vi "test TCX read (installed 71).vi"() -> ()   [LabVIEW 2011] (continued)
xmlns=\"http://www.garmin.com/xmlschemas/ActivityExtension/v2\"><Watts>70</Watts></TPX></Extensions></Trackpoint><Trackpoint><Time>2008-03-03T23:11:28Z</Time><Position><LatitudeDegrees>35.863362</LatitudeDegrees><LongitudeDegrees>-78.899874</LongitudeDegrees></Position><AltitudeMeters>78.004</AltitudeMeters><DistanceMeters>14315.783</DistanceMeters><Cadence>88</Cadence><Extensions><TPX xmlns=\"http://www.garmin.com/xmlschemas/ActivityExtension/v2\"><Watts>106</Watts></TPX></Extensions></Trackpoint><Trackpoint><Time>2008-03-03T23:11:29Z</Time><Position><LatitudeDegrees>35.863341</LatitudeDegrees><LongitudeDegrees>-78.900001</LongitudeDegrees></Position><AltitudeMeters>78.004</AltitudeMeters><DistanceMeters>14327.517</DistanceMeters><Cadence>89</Cadence><Extensions><TPX xmlns=\"http://www.garmin.com/xmlschemas/ActivityExtension/v2\"><Watts>108</Watts></TPX></Extensions></Trackpoint><Trackpoint><Time>2008-03-03T23:11:30Z</Time><Position><LatitudeDegrees>35.863322</LatitudeDegrees><LongitudeDegrees>-78.900129</LongitudeDegrees></Position><AltitudeMeters>77.523</AltitudeMeters><DistanceMeters>14339.211</DistanceMeters><Cadence>89</Cadence><Extensions><TPX xmlns=\"http://www.garmin.com/xmlschemas/ActivityExtension/v2\"><Watts>84</Watts></TPX></Extensions></Trackpoint><Trackpoint><Time>2008-03-03T23:11:31Z</Time><Position><LatitudeDegrees>35.863302</LatitudeDegrees><LongitudeDegrees>-78.900256</LongitudeDegrees></Position><AltitudeMeters>76.562</AltitudeMeters><DistanceMeters>14350.880</DistanceMeters><Cadence>88</Cadence><Extensions><TPX xmlns=\"http://www.garmin.com/xmlschemas/ActivityExtension/v2\"><Watts>71</Watts></TPX></Extensions></Trackpoint><Trackpoint><Time>2008-03-03T23:11:32Z</Time><Position><LatitudeDegrees>35.863280</LatitudeDegrees><LongitudeDegrees>-78.900379</LongitudeDegrees></Position><AltitudeMeters>76.562</AltitudeMeters><DistanceMeters>14362.324</DistanceMeters><Cadence>87</Cadence><Extensions><TPX xmlns=\"http://www.garmin.com/xmlschemas/ActivityExtension/v2\"><Watts>71</Watts></TPX></Extensions></Trackpoint><Trackpoint><Time>2008-03-03T23:11:33Z</Time><Position><LatitudeDegrees>35.863260</LatitudeDegrees><LongitudeDegrees>-78.900502</LongitudeDegrees></Position><AltitudeMeters>75.601</AltitudeMeters><DistanceMeters>14373.616</DistanceMeters><Cadence>86</Cadence><Extensions><TPX xmlns=\"http://www.garmin.com/xmlschemas/ActivityExtension/v2\"><Watts>86</Watts></TPX></Extensions></Trackpoint><Trackpoint><Time>2008-03-03T23:11:34Z</Time><Position><LatitudeDegrees>35.863238</LatitudeDegrees><LongitudeDegrees>-78.900622</LongitudeDegrees></Position><AltitudeMeters>75.601</AltitudeMeters><DistanceMeters>14384.671</DistanceMeters><Cadence>84</Cadence><Extensions><TPX xmlns=\"http://www.garmin.com/xmlschemas/ActivityExtension/v2\"><Watts>96</Watts></TPX></Extensions></Trackpoint><Trackpoint><Time>2008-03-03T23:11:35Z</Time><Position><LatitudeDegrees>35.863220</LatitudeDegrees><LongitudeDegrees>-78.900737</LongitudeDegrees></Position><AltitudeMeters>76.081</AltitudeMeters><DistanceMeters>14395.224</DistanceMeters><Cadence>81</Cadence><Extensions><TPX xmlns=\"http://www.garmin.com/xmlschemas/ActivityExtension/v2\"><Watts>97</Watts></TPX></Extensions></Trackpoint><Trackpoint><Time>2008-03-03T23:11:36Z</Time><Position><LatitudeDegrees>35.863205</LatitudeDegrees><LongitudeDegrees>-78.900847</LongitudeDegrees></Position><AltitudeMeters>75.601</AltitudeMeters><DistanceMeters>14405.182</DistanceMeters><Cadence>79</Cadence><Extensions><TPX xmlns=\"http://www.garmin.com/xmlschemas/ActivityExtension/v2\"><Watts>97</Watts></TPX></Extensions></Trackpoint><Trackpoint><Time>2008-03-03T23:11:37Z</Time><Position><LatitudeDegrees>35.863188</LatitudeDegrees><LongitudeDegrees>-78.900954</LongitudeDegrees></Position><AltitudeMeters>76.081</AltitudeMeters><DistanceMeters>14415.110</DistanceMeters><Cadence>75</Cadence><Extensions><TPX xmlns=\"http://www.garmin.com/xmlschemas/ActivityExtension/v2\"><Watts>109</Watts></TPX></Extensions></Trackpoint><Trackpoint><Time>2008-03-03T23:11:38Z</Time><Position><LatitudeDegrees>35.863172</LatitudeDegrees><LongitudeDegrees>-78.901058</LongitudeDegrees></Position><AltitudeMeters>76.081</AltitudeMeters><DistanceMeters>14424.662</DistanceMeters><Cadence>72</Cadence><Extensions><TPX xmlns=\"http://www.garmin.com/xmlschemas/ActivityExtension/v2\"><Watts>151</Watts></TPX></Extensions></Trackpoint><Trackpoint><Time>2008-03-03T23:11:39Z</Time><Position><LatitudeDegrees>35.863153</LatitudeDegrees><LongitudeDegrees>-78.901160</LongitudeDegrees></Position><AltitudeMeters>76.562</AltitudeMeters><DistanceMeters>14434.011</DistanceMeters><Cadence>72</Cadence><Extensions><TPX xmlns=\"http://www.garmin.com/xmlschemas/ActivityExtension/v2\"><Watts>152</Watts></TPX></Extensions></Trackpoint><Trackpoint><Time>2008-03-03T23:11:40Z</Time><Position><LatitudeDegrees>35.863133</LatitudeDegrees><LongitudeDegrees>-78.901258</LongitudeDegrees></Position><AltitudeMeters>77.043</AltitudeMeters><DistanceMeters>14443.188</DistanceMeters><Cadence>70</Cadence><Extensions><TPX xmlns=\"http://www.garmin.com/xmlschemas/ActivityExtension/v2\"><Watts>227</Watts></TPX></Extensions></Trackpoint><Trackpoint><Time>2008-03-03T23:11:41Z</Time><Position><LatitudeDegrees>35.863114</LatitudeDegrees><LongitudeDegrees>-78.901354</LongitudeDegrees></Position><AltitudeMeters>77.043</AltitudeMeters><DistanceMeters>14452.078</DistanceMeters><Cadence>68</Cadence><Extensions><TPX xmlns=\"http://www.garmin.com/xmlschemas/ActivityExtension/v2\"><Watts>274</Watts></TPX></Extensions></Trackpoint><Trackpoint><Time>2008-03-03T23:11:42Z</Time><Position><LatitudeDegrees>35.863093</LatitudeDegrees><LongitudeDegrees>-78.901448</LongitudeDegrees></Position><AltitudeMeters>77.043</AltitudeMeters><DistanceMeters>14460.851</DistanceMeters><Cadence>67</Cadence><Extensions><TPX xmlns=\"http://www.garmin.com/xmlschemas/ActivityExtension/v2\"><Watts>260</Watts></TPX></Extensions></Trackpoint><Trackpoint><Time>2008-03-03T23:11:43Z</Time><Position><LatitudeDegrees>35.863073</LatitudeDegrees><LongitudeDegrees>-78.901541</LongitudeDegrees></Position><AltitudeMeters>77.043</AltitudeMeters><DistanceMeters>14469.592</DistanceMeters><Cadence>67</Cadence><Extensions><TPX xmlns=\"http://www.garmin.com/xmlschemas/ActivityExtension/v2\"><Watts>261</Watts></TPX></Extensions></Trackpoint><Trackpoint><Time>2008-03-03T23:11:44Z</Time><Position><LatitudeDegrees>35.863051</LatitudeDegrees><LongitudeDegrees>-78.901635</LongitudeDegrees></Position><AltitudeMeters>77.043</AltitudeMeters><DistanceMeters>14478.395</DistanceMeters><Cadence>66</Cadence><Extensions><TPX xmlns=\"http://www.garmin.com/xmlschemas/ActivityExtension/v2\"><Watts>229</Watts></TPX></Extensions></Trackpoint><Trackpoint><Time>2008-03-03T23:11:45Z</Time><Position><LatitudeDegrees>35.863029</LatitudeDegrees><LongitudeDegrees>-78.901729</LongitudeDegrees></Position><AltitudeMeters>78.004</AltitudeMeters><DistanceMeters>14487.213</DistanceMeters><Cadence>67</Cadence><Extensions><TPX xmlns=\"http://www.garmin.com/xmlschemas/ActivityExtension/v2\"><Watts>209</Watts></TPX></Extensions></Trackpoint><Trackpoint><Time>2008-03-03T23:11:46Z</Time><Position><LatitudeDegrees>35.863005</LatitudeDegrees><LongitudeDegrees>-78.901822</LongitudeDegrees></Position><AltitudeMeters>78.004</AltitudeMeters><DistanceMeters>14496.032</DistanceMeters><Cadence>67</Cadence><Extensions><TPX xmlns=\"http://www.garmin.com/xmlschemas/ActivityExtension/v2\"><Watts>201</Watts></TPX></Extensions></Trackpoint><Trackpoint><Time>2008-03-03T23:11:47Z</Time><Position><LatitudeDegrees>35.862982</LatitudeDegrees><LongitudeDegrees>-78.901916</LongitudeDegrees></Position><AltitudeMeters>78.004</AltitudeMeters><DistanceMeters>14504.937</DistanceMeters><Cadence>68</Cadence><Extensions><TPX xmlns=\"http://www.garmin.com/xmlschemas/ActivityExtension/v2\"><Watts>202</Watts></TPX></Extensions></Trackpoint><Trackpoint><Time>2008-03-03T23:11:48Z</Time><Position><LatitudeDegrees>35.862958</LatitudeDegrees><LongitudeDegrees>-78.902011</LongitudeDegrees></Position><AltitudeMeters>77.523</AltitudeMeters><DistanceMeters>14513.910</DistanceMeters><Cadence>69</Cadence><Extensions><TPX xmlns=\"http://www.garmin.com/xmlschemas/ActivityExtension/v2\"><Watts>197</Watts></TPX></Extensions></Trackpoint><Trackpoint><Time>2008-03-03T23:11:49Z</Time><Position><LatitudeDegrees>35.862929</LatitudeDegrees><LongitudeDegrees>-78.902105</LongitudeDegrees></Position><AltitudeMeters>77.523</AltitudeMeters><DistanceMeters>14523.009</DistanceMeters><Cadence>69</Cadence><Extensions><TPX xmlns=\"http://www.garmin.com/xmlschemas/ActivityExtension/v2\"><Watts>197</Watts></TPX></Extensions></Trackpoint><Trackpoint><Time>2008-03-03T23:11:50Z</Time><Position><LatitudeDegrees>35.862900</LatitudeDegrees><LongitudeDegrees>-78.902200</LongitudeDegrees></Position><AltitudeMeters>78.004</AltitudeMeters><DistanceMeters>14532.178</DistanceMeters><Cadence>69</Cadence><Extensions><TPX xmlns=\"http://www.garmin.com/xmlschemas/ActivityExtension/v2\"><Watts>192</Watts></TPX></Extensions></Trackpoint><Trackpoint><Time>2008-03-03T23:11:51Z</Time><Position><LatitudeDegrees>35.862869</LatitudeDegrees><LongitudeDegrees>-78.902294</LongitudeDegrees></Position><AltitudeMeters>77.043</AltitudeMeters><DistanceMeters>14541.325</DistanceMeters><Cadence>69</Cadence><Extensions><TPX xmlns=\"http://www.garmin.com/xmlschemas/ActivityExtension/v2\"><Watts>192</Watts></TPX></Extensions></Trackpoint><Trackpoint><Time>2008-03-03T23:11:52Z</Time><Position><LatitudeDegrees>35.862839</LatitudeDegrees><LongitudeDegrees>-78.902389</LongitudeDegrees></Position><AltitudeMeters>76.562</AltitudeMeters><DistanceMeters>14550.554</DistanceMeters><Cadence>70</Cadence><Extensions><TPX xmlns=\"http://www.garmin.com/xmlschemas/ActivityExtension/v2\"><Watts>177</Watts></TPX></Extensions></Trackpoint><Trackpoint><Time>2008-03-03T23:11:53Z</Time><Position><LatitudeDegrees>35.862807</LatitudeDegrees><LongitudeDegrees>-78.902486</LongitudeDegrees></Position><AltitudeMeters>77.043</AltitudeMeters><DistanceMeters>14559.941</DistanceMeters><Cadence>71</Cadence><Extensions><TPX xmlns=\"http://www.garmin.com/xmlschemas/ActivityExtension/v2\"><Watts>164</Watts></TPX></Extensions></Trackpoint><Trackpoint><Time>2008-03-03T23:11:54Z</Time><Position><LatitudeDegrees>35.862774</LatitudeDegrees><LongitudeDegrees>-78.902581</LongitudeDegrees></Position><AltitudeMeters>76.562</AltitudeMeters><DistanceMeters>14569.321</DistanceMeters><Cadence>71</Cadence><Extensions><TPX xmlns=\"http://www.garmin.com/xmlschemas/ActivityExtension/v2\"><Watts>150</Watts></TPX></Extensions></Trackpoint><Trackpoint><Time>2008-03-03T23:11:55Z</Time><Position><LatitudeDegrees>35.862742</LatitudeDegrees><LongitudeDegrees>-78.902678</LongitudeDegrees></Position><AltitudeMeters>76.562</AltitudeMeters><DistanceMeters>14578.787</DistanceMeters><Cadence>72</Cadence><Extensions><TPX xmlns=\"http://www.garmin.com/xmlschemas/ActivityExtension/v2\"><Watts>137</Watts></TPX></Extensions></Trackpoint><Trackpoint><Time>2008-03-03T23:11:56Z</Time><Position><LatitudeDegrees>35.862709</LatitudeDegrees><LongitudeDegrees>-78.902777</LongitudeDegrees></Position><AltitudeMeters>76.081</AltitudeMeters><DistanceMeters>14588.439</DistanceMeters><Cadence>72</Cadence><Extensions><TPX xmlns=\"http://www.garmin.com/xmlschemas/ActivityExtension/v2\"><Watts>136</Watts></TPX></Extensions></Trackpoint><Trackpoint><Time>2008-03-03T23:11:57Z</Time><Position><LatitudeDegrees>35.862676</LatitudeDegrees><LongitudeDegrees>-78.902876</LongitudeDegrees></Position><AltitudeMeters>76.081</AltitudeMeters><DistanceMeters>14598.146</DistanceMeters><Cadence>74</Cadence><Extensions><TPX xmlns=\"http://www.garmin.com/xmlschemas/ActivityExtension/v2\"><Watts>129</Watts></TPX></Extensions></Trackpoint><Trackpoint><Time>2008-03-03T23:11:58Z</Time><Position><LatitudeDegrees>35.862642</LatitudeDegrees><LongitudeDegrees>-78.902977</LongitudeDegrees></Position><AltitudeMeters>76.081</AltitudeMeters><DistanceMeters>14607.972</DistanceMeters><Cadence>74</Cadence><Extensions><TPX xmlns=\"http://www.garmin.com/xmlschemas/ActivityExtension/v2\"><Watts>128</Watts></TPX></Extensions></Trackpoint><Trackpoint><Time>2008-03-03T23:11:59Z</Time><Position><LatitudeDegrees>35.862609</LatitudeDegrees><LongitudeDegrees>-78.903079</LongitudeDegrees></Position><AltitudeMeters>75.601</AltitudeMeters><DistanceMeters>14617.938</DistanceMeters><Cadence>76</Cadence><Extensions><TPX xmlns=\"http://www.garmin.com/xmlschemas/ActivityExtension/v2\"><Watts>102</Watts></TPX></Extensions></Trackpoint><Trackpoint><Time>2008-03-03T23:12:00Z</Time><Position><LatitudeDegrees>35.862574</LatitudeDegrees><LongitudeDegrees>-78.903183</LongitudeDegrees></Position><AltitudeMeters>75.601</AltitudeMeters><DistanceMeters>14628.073</DistanceMeters><Cadence>77</Cadence><Extensions><TPX xmlns=\"http://www.garmin.com/xmlschemas/ActivityExtension/v2\"><Watts>87</Watts></TPX></Extensions></Trackpoint><Trackpoint><Time>2008-03-03T23:12:01Z</Time><Position><LatitudeDegrees>35.862540</LatitudeDegrees><LongitudeDegrees>-78.903288</LongitudeDegrees></Position><AltitudeMeters>75.601</AltitudeMeters><DistanceMeters>14638.298</DistanceMeters><Cadence>77</Cadence><Extensions><TPX xmlns=\"http://www.garmin.com/xmlschemas/ActivityExtension/v2\"><Watts>87</Watts></TPX></Extensions></Trackpoint><Trackpoint><Time>2008-03-03T23:12:02Z</Time><Position><LatitudeDegrees>35.862505</LatitudeDegrees><LongitudeDegrees>-78.903394</LongitudeDegrees></Position><AltitudeMeters>75.601</AltitudeMeters><DistanceMeters>14648.685</DistanceMeters><Cadence>78</Cadence><Extensions><TPX xmlns=\"http://www.garmin.com/xmlschemas/ActivityExtension/v2\"><Watts>87</Watts></TPX></Extensions></Trackpoint><Trackpoint><Time>2008-03-03T23:12:03Z</Time><Position><LatitudeDegrees>35.862470</LatitudeDegrees><LongitudeDegrees>-78.903503</LongitudeDegrees></Position><AltitudeMeters>75.120</AltitudeMeters><DistanceMeters>14659.182</DistanceMeters><Cadence>79</Cadence><Extensions><TPX xmlns=\"http://www.garmin.com/xmlschemas/ActivityExtension/v2\"><Watts>87</Watts></TPX></Extensions></Trackpoint><Trackpoint><Time>2008-03-03T23:12:04Z</Time><Position><LatitudeDegrees>35.862435</LatitudeDegrees><LongitudeDegrees>-78.903612</LongitudeDegrees></Position><AltitudeMeters>74.640</AltitudeMeters><DistanceMeters>14669.802</DistanceMeters><Cadence>80</Cadence><Extensions><TPX xmlns=\"http://www.garmin.com/xmlschemas/ActivityExtension/v2\"><Watts>93</Watts></TPX></Extensions></Trackpoint><Trackpoint><Time>2008-03-03T23:12:05Z</Time><Position><LatitudeDegrees>35.862398</LatitudeDegrees><LongitudeDegrees>-78.903722</LongitudeDegrees></Position><AltitudeMeters>73.678</AltitudeMeters><DistanceMeters>14680.509</DistanceMeters><Cadence>81</Cadence><Extensions><TPX xmlns=\"http://www.garmin.com/xmlschemas/ActivityExtension/v2\"><Watts>94</Watts></TPX></Extensions></Trackpoint><Trackpoint><Time>2008-03-03T23:12:06Z</Time><Position><LatitudeDegrees>35.862362</LatitudeDegrees><LongitudeDegrees>-78.903832</LongitudeDegrees></Position><AltitudeMeters>73.198</AltitudeMeters><DistanceMeters>14691.294</DistanceMeters><Cadence>82</Cadence><Extensions><TPX xmlns=\"http://www.garmin.com/xmlschemas/ActivityExtension/v2\"><Watts>92</Watts></TPX></Extensions></Trackpoint><Trackpoint><Time>2008-03-03T23:12:07Z</Time><Position><LatitudeDegrees>35.862326</LatitudeDegrees><LongitudeDegrees>-78.903942</LongitudeDegrees></Position><AltitudeMeters>73.198</AltitudeMeters><DistanceMeters>14702.009</DistanceMeters><Cadence>81</Cadence><Extensions><TPX xmlns=\"http://www.garmin.com/xmlschemas/ActivityExtension/v2\"><Watts>97</Watts></TPX></Extensions></Trackpoint><Trackpoint><Time>2008-03-03T23:12:08Z</Time><Position><LatitudeDegrees>35.862289</LatitudeDegrees><LongitudeDegrees>-78.904050</LongitudeDegrees></Position><AltitudeMeters>73.678</AltitudeMeters><DistanceMeters>14712.588</DistanceMeters><Cadence>80</Cadence><Extensions><TPX xmlns=\"http://www.garmin.com/xmlschemas/ActivityExtension/v2\"><Watts>97</Watts></TPX></Extensions></Trackpoint><Trackpoint><Time>2008-03-03T23:12:09Z</Time><Position><LatitudeDegrees>35.862253</LatitudeDegrees><LongitudeDegrees>-78.904157</LongitudeDegrees></Position><AltitudeMeters>73.198</AltitudeMeters><DistanceMeters>14723.039</DistanceMeters><Cadence>79</Cadence><Extensions><TPX xmlns=\"http://www.garmin.com/xmlschemas/ActivityExtension/v2\"><Watts>125</Watts></TPX></Extensions></Trackpoint><Trackpoint><Time>2008-03-03T23:12:10Z</Time><Position><LatitudeDegrees>35.862219</LatitudeDegrees><LongitudeDegrees>-78.904263</LongitudeDegrees></Position><AltitudeMeters>73.678</AltitudeMeters><DistanceMeters>14733.320</DistanceMeters><Cadence>79</Cadence><Extensions><TPX xmlns=\"http://www.garmin.com/xmlschemas/ActivityExtension/v2\"><Watts>124</Watts></TPX></Extensions></Trackpoint><Trackpoint><Time>2008-03-03T23:12:11Z</Time><Position><LatitudeDegrees>35.862188</LatitudeDegrees><LongitudeDegrees>-78.904368</LongitudeDegrees></Position><AltitudeMeters>73.678</AltitudeMeters><DistanceMeters>14743.404</DistanceMeters><Cadence>77</Cadence><Extensions><TPX xmlns=\"http://www.garmin.com/xmlschemas/ActivityExtension/v2\"><Watts>144</Watts></TPX></Extensions></Trackpoint><Trackpoint><Time>2008-03-03T23:12:12Z</Time><Position><LatitudeDegrees>35.862162</LatitudeDegrees><LongitudeDegrees>-78.904473</LongitudeDegrees></Position><AltitudeMeters>74.159</AltitudeMeters><DistanceMeters>14753.264</DistanceMeters><Cadence>73</Cadence><Extensions><TPX xmlns=\"http://www.garmin.com/xmlschemas/ActivityExtension/v2\"><Watts>176</Watts></TPX></Extensions></Trackpoint><Trackpoint><Time>2008-03-03T23:12:13Z</Time><Position><LatitudeDegrees>35.862142</LatitudeDegrees><LongitudeDegrees>-78.904576</LongitudeDegrees></Position><AltitudeMeters>74.640</AltitudeMeters><DistanceMeters>14762.778</DistanceMeters><Cadence>73</Cadence><Extensions><TPX xmlns=\"http://www.garmin.com/xmlschemas/ActivityExtension/v2\"><Watts>176</Watts></TPX></Extensions></Trackpoint><Trackpoint><Time>2008-03-03T23:12:14Z</Time><Position><LatitudeDegrees>35.862129</LatitudeDegrees><LongitudeDegrees>-78.904676</LongitudeDegrees></Position><AltitudeMeters>75.120</AltitudeMeters><DistanceMeters>14771.976</DistanceMeters><Cadence>69</Cadence><Extensions><TPX xmlns=\"http://www.garmin.com/xmlschemas/ActivityExtension/v2\"><Watts>178</Watts></TPX></Extensions></Trackpoint><Trackpoint><Time>2008-03-03T23:12:15Z</Time><Position><LatitudeDegrees>35.862125</LatitudeDegrees><LongitudeDegrees>-78.904774</LongitudeDegrees></Position><AltitudeMeters>75.120</AltitudeMeters><DistanceMeters>14780.801</DistanceMeters><Cadence>67</Cadence><Extensions><TPX xmlns=\"http://www.garmin.com/xmlschemas/ActivityExtension/v2\"><Watts>180</Watts></TPX></Extensions></Trackpoint><Trackpoint><Time>2008-03-03T23:12:16Z</Time><Position><LatitudeDegrees>35.862130</LatitudeDegrees><LongitudeDegrees>-78.904870</LongitudeDegrees></Position><AltitudeMeters>75.601</AltitudeMeters><DistanceMeters>14789.530</DistanceMeters><Cadence>66</Cadence><Extensions><TPX xmlns=\"http://www.garmin.com/xmlschemas/ActivityExtension/v2\"><Watts>190</Watts></TPX></Extensions></Trackpoint><Trackpoint><Time>2008-03-03T23:12:17Z</Time><Position><LatitudeDegrees>35.862142</LatitudeDegrees><LongitudeDegrees>-78.904963</LongitudeDegrees></Position><AltitudeMeters>75.601</AltitudeMeters><DistanceMeters>14797.981</DistanceMeters><Cadence>66</Cadence><Extensions><TPX xmlns=\"http://www.garmin.com/xmlschemas/ActivityExtension/v2\"><Watts>192</Watts></TPX></Extensions></Trackpoint><Trackpoint><Time>2008-03-03T23:12:18Z</Time><Position><LatitudeDegrees>35.862161</LatitudeDegrees><LongitudeDegrees>-78.905054</LongitudeDegrees></Position><AltitudeMeters>75.601</AltitudeMeters><DistanceMeters>14806.480</DistanceMeters><Cadence>66</Cadence><Extensions><TPX xmlns=\"http://www.garmin.com/xmlschemas/ActivityExtension/v2\"><Watts>191</Watts></TPX></Extensions></Trackpoint><Trackpoint><Time>2008-03-03T23:12:19Z</Time><Position><LatitudeDegrees>35.862188</LatitudeDegrees><LongitudeDegrees>-78.905144</LongitudeDegrees></Position><AltitudeMeters>74.640</AltitudeMeters><DistanceMeters>14815.028</DistanceMeters><Cadence>66</Cadence><Extensions><TPX xmlns=\"http://www.garmin.com/xmlschemas/ActivityExtension/v2\"><Watts>185</Watts></TPX></Extensions></Trackpoint><Trackpoint><Time>2008-03-03T23:12:20Z</Time><Position><LatitudeDegrees>35.862220</LatitudeDegrees><LongitudeDegrees>-78.905230</LongitudeDegrees></Position><AltitudeMeters>74.640</AltitudeMeters><DistanceMeters>14823.684</DistanceMeters><Cadence>66</Cadence><Extensions><TPX xmlns=\"http://www.garmin.com/xmlschemas/ActivityExtension/v2\"><Watts>183</Watts></TPX></Extensions></Trackpoint><Trackpoint><Time>2008-03-03T23:12:21Z</Time><Position><LatitudeDegrees>35.862256</LatitudeDegrees><LongitudeDegrees>-78.905316</LongitudeDegrees></Position><AltitudeMeters>74.159</AltitudeMeters><DistanceMeters>14832.372</DistanceMeters><Cadence>67</Cadence><Extensions><TPX xmlns=\"http://www.garmin.com/xmlschemas/ActivityExtension/v2\"><Watts>179</Watts></TPX></Extensions></Trackpoint><Trackpoint><Time>2008-03-03T23:12:22Z</Time><Position><LatitudeDegrees>35.862293</LatitudeDegrees><LongitudeDegrees>-78.905401</LongitudeDegrees></Position><AltitudeMeters>74.159</AltitudeMeters><DistanceMeters>14841.090</DistanceMeters><Cadence>67</Cadence><Extensions><TPX xmlns=\"http://www.garmin.com/xmlschemas/ActivityExtension/v2\"><Watts>168</Watts></TPX></Extensions></Trackpoint><Trackpoint><Time>2008-03-03T23:12:23Z</Time><Position><LatitudeDegrees>35.862330</LatitudeDegrees><LongitudeDegrees>-78.905486</LongitudeDegrees></Position><AltitudeMeters>74.159</AltitudeMeters><DistanceMeters>14849.768</DistanceMeters><Cadence>66</Cadence><Extensions><TPX xmlns=\"http://www.garmin.com/xmlschemas/ActivityExtension/v2\"><Watts>170</Watts></TPX></Extensions></Trackpoint><Trackpoint><Time>2008-03-03T23:12:24Z</Time><Position><LatitudeDegrees>35.862367</LatitudeDegrees><LongitudeDegrees>-78.905570</LongitudeDegrees></Position><AltitudeMeters>74.159</AltitudeMeters><DistanceMeters>14858.395</DistanceMeters><Cadence>66</Cadence><Extensions><TPX xmlns=\"http://www.garmin.com/xmlschemas/ActivityExtension/v2\"><Watts>173</Watts></TPX></Extensions></Trackpoint><Trackpoint><Time>2008-03-03T23:12:25Z</Time><Position><LatitudeDegrees>35.862405</LatitudeDegrees><LongitudeDegrees>-78.905651</LongitudeDegrees></Position><AltitudeMeters>74.640</AltitudeMeters><DistanceMeters>14866.879</DistanceMeters><Cadence>65</Cadence><Extensions><TPX xmlns=\"http://www.garmin.com/xmlschemas/ActivityExtension/v2\"><Watts>169</Watts></TPX></Extensions></Trackpoint><Trackpoint><Time>2008-03-03T23:12:26Z</Time><Position><LatitudeDegrees>35.862443</LatitudeDegrees><LongitudeDegrees>-78.905731</LongitudeDegrees></Position><AltitudeMeters>74.640</AltitudeMeters><DistanceMeters>14875.242</DistanceMeters><Cadence>68</Cadence><Extensions><TPX xmlns=\"http://www.garmin.com/xmlschemas/ActivityExtension/v2\"><Watts>164</Watts></TPX></Extensions></Trackpoint><Trackpoint><Time>2008-03-03T23:12:27Z</Time><Position><LatitudeDegrees>35.862480</LatitudeDegrees><LongitudeDegrees>-78.905811</LongitudeDegrees></Position><AltitudeMeters>74.640</AltitudeMeters><DistanceMeters>14883.440</DistanceMeters><Cadence>76</Cadence><Extensions><TPX xmlns=\"http://www.garmin.com/xmlschemas/ActivityExtension/v2\"><Watts>171</Watts></TPX></Extensions></Trackpoint><Trackpoint><Time>2008-03-03T23:12:28Z</Time><Position><LatitudeDegrees>35.862514</LatitudeDegrees><LongitudeDegrees>-78.905888</LongitudeDegrees></Position><AltitudeMeters>75.120</AltitudeMeters><DistanceMeters>14891.395</DistanceMeters><Cadence>74</Cadence><Extensions><TPX xmlns=\"http://www.garmin.com/xmlschemas/ActivityExtension/v2\"><Watts>183</Watts></TPX></Extensions></Trackpoint><Trackpoint><Time>2008-03-03T23:12:29Z</Time><Position><LatitudeDegrees>35.862548</LatitudeDegrees><LongitudeDegrees>-78.905964</LongitudeDegrees></Position><AltitudeMeters>75.120</AltitudeMeters><DistanceMeters>14899.225</DistanceMeters><Cadence>72</Cadence><Extensions><TPX xmlns=\"http://www.garmin.com/xmlschemas/ActivityExtension/v2\"><Watts>260</Watts></TPX></Extensions></Trackpoint><Trackpoint><Time>2008-03-03T23:12:30Z</Time><Position><LatitudeDegrees>35.862580</LatitudeDegrees><LongitudeDegrees>-78.906040</LongitudeDegrees></Position><AltitudeMeters>75.601</AltitudeMeters><DistanceMeters>14906.950</DistanceMeters><Cadence>72</Cadence><Extensions><TPX xmlns=\"http://www.garmin.com/xmlschemas/ActivityExtension/v2\"><Watts>302</Watts></TPX></Extensions></Trackpoint><Trackpoint><Time>2008-03-03T23:12:31Z</Time><Position><LatitudeDegrees>35.862613</LatitudeDegrees><LongitudeDegrees>-78.906115</LongitudeDegrees></Position><AltitudeMeters>76.081</AltitudeMeters><DistanceMeters>14914.627</DistanceMeters><Cadence>72</Cadence><Extensions><TPX xmlns=\"http://www.garmin.com/xmlschemas/ActivityExtension/v2\"><Watts>337</Watts></TPX></Extensions></Trackpoint><Trackpoint><Time>2008-03-03T23:12:32Z</Time><Position><LatitudeDegrees>35.862646</LatitudeDegrees><LongitudeDegrees>-78.906190</LongitudeDegrees></Position><AltitudeMeters>76.081</AltitudeMeters><DistanceMeters>14922.329</DistanceMeters><Cadence>72</Cadence><Extensions><TPX xmlns=\"http://www.garmin.com/xmlschemas/ActivityExtension/v2\"><Watts>348</Watts></TPX></Extensions></Trackpoint><Trackpoint><Time>2008-03-03T23:12:33Z</Time><Position><LatitudeDegrees>35.862679</LatitudeDegrees><LongitudeDegrees>-78.906265</LongitudeDegrees></Position><AltitudeMeters>76.081</AltitudeMeters><DistanceMeters>14930.017</DistanceMeters><Cadence>72</Cadence><Extensions><TPX xmlns=\"http://www.garmin.com/xmlschemas/ActivityExtension/v2\"><Watts>346</Watts></TPX></Extensions></Trackpoint><Trackpoint><Time>2008-03-03T23:12:34Z</Time><Position><LatitudeDegrees>35.862711</LatitudeDegrees><LongitudeDegrees>-78.906340</LongitudeDegrees></Position><AltitudeMeters>76.562</AltitudeMeters><DistanceMeters>14937.709</DistanceMeters><Cadence>71</Cadence><Extensions><TPX xmlns=\"http://www.garmin.com/xmlschemas/ActivityExtension/v2\"><Watts>332</Watts></TPX></Extensions></Trackpoint><Trackpoint><Time>2008-03-03T23:12:35Z</Time><Position><LatitudeDegrees>35.862745</LatitudeDegrees><LongitudeDegrees>-78.906415</LongitudeDegrees></Position><AltitudeMeters>76.562</AltitudeMeters><DistanceMeters>14945.422</DistanceMeters><Cadence>71</Cadence><Extensions><TPX xmlns=\"http://www.garmin.com/xmlschemas/ActivityExtension/v2\"><Watts>331</Watts></TPX></Extensions></Trackpoint><Trackpoint><Time>2008-03-03T23:12:36Z</Time><Position><LatitudeDegrees>35.862779</LatitudeDegrees><LongitudeDegrees>-78.906490</LongitudeDegrees></Position><AltitudeMeters>77.043</AltitudeMeters><DistanceMeters>14953.136</DistanceMeters><Cadence>71</Cadence><Extensions><TPX xmlns=\"http://www.garmin.com/xmlschemas/ActivityExtension/v2\"><Watts>284</Watts></TPX></Extensions></Trackpoint><Trackpoint><Time>2008-03-03T23:12:37Z</Time><Position><LatitudeDegrees>35.862811</LatitudeDegrees><LongitudeDegrees>-78.906565</LongitudeDegrees></Position><AltitudeMeters>77.043</AltitudeMeters><DistanceMeters>14960.813</DistanceMeters><Cadence>71</Cadence><Extensions><TPX xmlns=\"http://www.garmin.com/xmlschemas/ActivityExtension/v2\"><Watts>233</Watts></TPX></Extensions></Trackpoint><Trackpoint><Time>2008-03-03T23:12:38Z</Time><Position><LatitudeDegrees>35.862843</LatitudeDegrees><LongitudeDegrees>-78.906641</LongitudeDegrees></Position><AltitudeMeters>77.523</AltitudeMeters><DistanceMeters>14968.545</DistanceMeters><Cadence>71</Cadence><Extensions><TPX xmlns=\"http://www.garmin.com/xmlschemas/ActivityExtension/v2\"><Watts>206</Watts></TPX></Extensions></Trackpoint><Trackpoint><Time>2008-03-03T23:12:39Z</Time><Position><LatitudeDegrees>35.862875</LatitudeDegrees><LongitudeDegrees>-78.906718</LongitudeDegrees></Position><AltitudeMeters>77.523</AltitudeMeters><DistanceMeters>14976.333</DistanceMeters><Cadence>72</Cadence><Extensions><TPX xmlns=\"http://www.garmin.com/xmlschemas/ActivityExtension/v2\"><Watts>140</Watts></TPX></Extensions></Trackpoint><Trackpoint><Time>2008-03-03T23:12:40Z</Time><Position><LatitudeDegrees>35.862907</LatitudeDegrees><LongitudeDegrees>-78.906796</LongitudeDegrees></Position><AltitudeMeters>77.523</AltitudeMeters><DistanceMeters>14984.246</DistanceMeters><Cadence>72</Cadence><Extensions><TPX xmlns=\"http://www.garmin.com/xmlschemas/ActivityExtension/v2\"><Watts>140</Watts></TPX></Extensions></Trackpoint><Trackpoint><Time>2008-03-03T23:12:41Z</Time><Position><LatitudeDegrees>35.862939</LatitudeDegrees><LongitudeDegrees>-78.906876</LongitudeDegrees></Position><AltitudeMeters>77.523</AltitudeMeters><DistanceMeters>14992.344</DistanceMeters><Cadence>74</Cadence><Extensions><TPX xmlns=\"http://www.garmin.com/xmlschemas/ActivityExtension/v2\"><Watts>133</Watts></TPX></Extensions></Trackpoint><Trackpoint><Time>2008-03-03T23:12:42Z</Time><Position><LatitudeDegrees>35.862969</LatitudeDegrees><LongitudeDegrees>-78.906960</LongitudeDegrees></Position><AltitudeMeters>77.043</AltitudeMeters><DistanceMeters>15000.614</DistanceMeters><Cadence>77</Cadence><Extensions><TPX xmlns=\"http://www.garmin.com/xmlschemas/ActivityExtension/v2\"><Watts>75</Watts></TPX></Extensions></Trackpoint><Trackpoint><Time>2008-03-03T23:12:43Z</Time><Position><LatitudeDegrees>35.862997</LatitudeDegrees><LongitudeDegrees>-78.907046</LongitudeDegrees></Position><AltitudeMeters>77.043</AltitudeMeters><DistanceMeters>15009.035</DistanceMeters><Cadence>78</Cadence><Extensions><TPX xmlns=\"http://www.garmin.com/xmlschemas/ActivityExtension/v2\"><Watts>77</Watts></TPX></Extensions></Trackpoint><Trackpoint><Time>2008-03-03T23:12:44Z</Time><Position><LatitudeDegrees>35.863024</LatitudeDegrees><LongitudeDegrees>-78.907136</LongitudeDegrees></Position><AltitudeMeters>77.043</AltitudeMeters><DistanceMeters>15017.611</DistanceMeters><Cadence>79</Cadence><Extensions><TPX xmlns=\"http://www.garmin.com/xmlschemas/ActivityExtension/v2\"><Watts>72</Watts></TPX></Extensions></Trackpoint><Trackpoint><Time>2008-03-03T23:12:45Z</Time><Position><LatitudeDegrees>35.863049</LatitudeDegrees><LongitudeDegrees>-78.907228</LongitudeDegrees></Position><AltitudeMeters>76.562</AltitudeMeters><DistanceMeters>15026.392</DistanceMeters><Cadence>80</Cadence><Extensions><TPX xmlns=\"http://www.garmin.com/xmlschemas/ActivityExtension/v2\"><Watts>69</Watts></TPX></Extensions></Trackpoint><Trackpoint><Time>2008-03-03T23:12:46Z</Time><Position><LatitudeDegrees>35.863074</LatitudeDegrees><LongitudeDegrees>-78.907321</LongitudeDegrees></Position><AltitudeMeters>75.601</AltitudeMeters><DistanceMeters>15035.325</DistanceMeters><Cadence>84</Cadence><Extensions><TPX xmlns=\"http://www.garmin.com/xmlschemas/ActivityExtension/v2\"><Watts>68</Watts></TPX></Extensions></Trackpoint><Trackpoint><Time>2008-03-03T23:12:47Z</Time><Position><LatitudeDegrees>35.863103</LatitudeDegrees><LongitudeDegrees>-78.907416</LongitudeDegrees></Position><AltitudeMeters>75.120</AltitudeMeters><DistanceMeters>15044.475</DistanceMeters><Cadence>86</Cadence><Extensions><TPX xmlns=\"http://www.garmin.com/xmlschemas/ActivityExtension/v2\"><Watts>59</Watts></TPX></Extensions></Trackpoint><Trackpoint><Time>2008-03-03T23:12:48Z</Time><Position><LatitudeDegrees>35.863139</LatitudeDegrees><LongitudeDegrees>-78.907511</LongitudeDegrees></Position><AltitudeMeters>76.081</AltitudeMeters><DistanceMeters>15053.896</DistanceMeters><Cadence>88</Cadence><Extensions><TPX xmlns=\"http://www.garmin.com/xmlschemas/ActivityExtension/v2\"><Watts>57</Watts></TPX></Extensions></Trackpoint><Trackpoint><Time>2008-03-03T23:12:49Z</Time><Position><LatitudeDegrees>35.863174</LatitudeDegrees><LongitudeDegrees>-78.907608</LongitudeDegrees></Position><AltitudeMeters>75.120</AltitudeMeters><DistanceMeters>15063.466</DistanceMeters><Cadence>89</Cadence><Extensions><TPX xmlns=\"http://www.garmin.com/xmlschemas/ActivityExtension/v2\"><Watts>59</Watts></TPX></Extensions></Trackpoint><Trackpoint><Time>2008-03-03T23:12:50Z</Time><Position><LatitudeDegrees>35.863203</LatitudeDegrees><LongitudeDegrees>-78.907710</LongitudeDegrees></Position><AltitudeMeters>74.640</AltitudeMeters><DistanceMeters>15073.261</DistanceMeters><Cadence>87</Cadence><Extensions><TPX xmlns=\"http://www.garmin.com/xmlschemas/ActivityExtension/v2\"><Watts>61</Watts></TPX></Extensions></Trackpoint><Trackpoint><Time>2008-03-03T23:12:51Z</Time><Position><LatitudeDegrees>35.863233</LatitudeDegrees><LongitudeDegrees>-78.907813</LongitudeDegrees></Position><AltitudeMeters>74.159</AltitudeMeters><DistanceMeters>15083.226</DistanceMeters><Cadence>81</Cadence><Extensions><TPX xmlns=\"http://www.garmin.com/xmlschemas/ActivityExtension/v2\"><Watts>76</Watts></TPX></Extensions></Trackpoint><Trackpoint><Time>2008-03-03T23:12:52Z</Time><Position><LatitudeDegrees>35.863264</LatitudeDegrees><LongitudeDegrees>-78.907918</LongitudeDegrees></Position><AltitudeMeters>73.678</AltitudeMeters><DistanceMeters>15093.287</DistanceMeters><Cadence>82</Cadence><Extensions><TPX xmlns=\"http://www.garmin.com/xmlschemas/ActivityExtension/v2\"><Watts>81</Watts></TPX></Extensions></Trackpoint><Trackpoint><Time>2008-03-03T23:12:53Z</Time><Position><LatitudeDegrees>35.863293</LatitudeDegrees><LongitudeDegrees>-78.908025</LongitudeDegrees></Position><AltitudeMeters>73.198</AltitudeMeters><DistanceMeters>15103.444</DistanceMeters><Cadence>83</Cadence><Extensions><TPX xmlns=\"http://www.garmin.com/xmlschemas/ActivityExtension/v2\"><Watts>91</Watts></TPX></Extensions></Trackpoint><Trackpoint><Time>2008-03-03T23:12:54Z</Time><Position><LatitudeDegrees>35.863322</LatitudeDegrees><LongitudeDegrees>-78.908133</LongitudeDegrees></Position><AltitudeMeters>73.678</AltitudeMeters><DistanceMeters>15113.717</DistanceMeters><Cadence>84</Cadence><Extensions><TPX xmlns=\"http://www.garmin.com/xmlschemas/ActivityExtension/v2\"><Watts>90</Watts></TPX></Extensions></Trackpoint><Trackpoint><Time>2008-03-03T23:12:55Z</Time><Position><LatitudeDegrees>35.863350</LatitudeDegrees><LongitudeDegrees>-78.908243</LongitudeDegrees></Position><AltitudeMeters>73.678</AltitudeMeters><DistanceMeters>15124.105</DistanceMeters><Cadence>85</Cadence><Extensions><TPX xmlns=\"http://www.garmin.com/xmlschemas/ActivityExtension/v2\"><Watts>97</Watts></TPX></Extensions></Trackpoint><Trackpoint><Time>2008-03-03T23:12:56Z</Time><Position><LatitudeDegrees>35.863378</LatitudeDegrees><LongitudeDegrees>-78.908353</LongitudeDegrees></Position><AltitudeMeters>72.717</AltitudeMeters><DistanceMeters>15134.520</DistanceMeters><Cadence>85</Cadence><Extensions><TPX xmlns=\"http://www.garmin.com/xmlschemas/ActivityExtension/v2\"><Watts>115</Watts></TPX></Extensions></Trackpoint><Trackpoint><Time>2008-03-03T23:12:57Z</Time><Position><LatitudeDegrees>35.863403</LatitudeDegrees><LongitudeDegrees>-78.908464</LongitudeDegrees></Position><AltitudeMeters>73.198</AltitudeMeters><DistanceMeters>15144.966</DistanceMeters><Cadence>85</Cadence><Extensions><TPX xmlns=\"http://www.garmin.com/xmlschemas/ActivityExtension/v2\"><Watts>113</Watts></TPX></Extensions></Trackpoint><Trackpoint><Time>2008-03-03T23:12:58Z</Time><Position><LatitudeDegrees>35.863427</LatitudeDegrees><LongitudeDegrees>-78.908575</LongitudeDegrees></Position><AltitudeMeters>72.717</AltitudeMeters><DistanceMeters>15155.300</DistanceMeters><Cadence>84</Cadence><Extensions><TPX xmlns=\"http://www.garmin.com/xmlschemas/ActivityExtension/v2\"><Watts>140</Watts></TPX></Extensions></Trackpoint><Trackpoint><Time>2008-03-03T23:12:59Z</Time><Position><LatitudeDegrees>35.863450</LatitudeDegrees><LongitudeDegrees>-78.908685</LongitudeDegrees></Position><AltitudeMeters>72.717</AltitudeMeters><DistanceMeters>15165.539</DistanceMeters><Cadence>83</Cadence><Extensions><TPX xmlns=\"http://www.garmin.com/xmlschemas/ActivityExtension/v2\"><Watts>141</Watts></TPX></Extensions></Trackpoint><Trackpoint><Time>2008-03-03T23:13:00Z</Time><Position><LatitudeDegrees>35.863471</LatitudeDegrees><LongitudeDegrees>-78.908793</LongitudeDegrees></Position><AltitudeMeters>73.198</AltitudeMeters><DistanceMeters>15175.586</DistanceMeters><Cadence>81</Cadence><Extensions><TPX xmlns=\"http://www.garmin.com/xmlschemas/ActivityExtension/v2\"><Watts>129</Watts></TPX></Extensions></Trackpoint><Trackpoint><Time>2008-03-03T23:13:01Z</Time><Position><LatitudeDegrees>35.863491</LatitudeDegrees><LongitudeDegrees>-78.908899</LongitudeDegrees></Position><AltitudeMeters>73.198</AltitudeMeters><DistanceMeters>15185.383</DistanceMeters><Cadence>79</Cadence><Extensions><TPX xmlns=\"http://www.garmin.com/xmlschemas/ActivityExtension/v2\"><Watts>112</Watts></TPX></Extensions></Trackpoint><Trackpoint><Time>2008-03-03T23:13:02Z</Time><Position><LatitudeDegrees>35.863510</LatitudeDegrees><LongitudeDegrees>-78.909003</LongitudeDegrees></Position><AltitudeMeters>73.198</AltitudeMeters><DistanceMeters>15194.972</DistanceMeters><Cadence>78</Cadence><Extensions><TPX xmlns=\"http://www.garmin.com/xmlschemas/ActivityExtension/v2\"><Watts>112</Watts></TPX></Extensions></Trackpoint><Trackpoint><Time>2008-03-03T23:13:03Z</Time><Position><LatitudeDegrees>35.863529</LatitudeDegrees><LongitudeDegrees>-78.909104</LongitudeDegrees></Position><AltitudeMeters>73.198</AltitudeMeters><DistanceMeters>15204.387</DistanceMeters><Cadence>76</Cadence><Extensions><TPX xmlns=\"http://www.garmin.com/xmlschemas/ActivityExtension/v2\"><Watts>129</Watts></TPX></Extensions></Trackpoint><Trackpoint><Time>2008-03-03T23:13:04Z</Time><Position><LatitudeDegrees>35.863546</LatitudeDegrees><LongitudeDegrees>-78.909204</LongitudeDegrees></Position><AltitudeMeters>73.678</AltitudeMeters><DistanceMeters>15213.527</DistanceMeters><Cadence>73</Cadence><Extensions><TPX xmlns=\"http://www.garmin.com/xmlschemas/ActivityExtension/v2\"><Watts>155</Watts></TPX></Extensions></Trackpoint><Trackpoint><Time>2008-03-03T23:13:05Z</Time><Position><LatitudeDegrees>35.863560</LatitudeDegrees><LongitudeDegrees>-78.909300</LongitudeDegrees></Position><AltitudeMeters>73.678</AltitudeMeters><DistanceMeters>15222.367</DistanceMeters><Cadence>73</Cadence><Extensions><TPX xmlns=\"http://www.garmin.com/xmlschemas/ActivityExtension/v2\"><Watts>157</Watts></TPX></Extensions></Trackpoint><Trackpoint><Time>2008-03-03T23:13:06Z</Time><Position><LatitudeDegrees>35.863575</LatitudeDegrees><LongitudeDegrees>-78.909395</LongitudeDegrees></Position><AltitudeMeters>73.198</AltitudeMeters><DistanceMeters>15231.122</DistanceMeters><Cadence>72</Cadence><Extensions><TPX xmlns=\"http://www.garmin.com/xmlschemas/ActivityExtension/v2\"><Watts>190</Watts></TPX></Extensions></Trackpoint><Trackpoint><Time>2008-03-03T23:13:07Z</Time><Position><LatitudeDegrees>35.863592</LatitudeDegrees><LongitudeDegrees>-78.909491</LongitudeDegrees></Position><AltitudeMeters>73.198</AltitudeMeters><DistanceMeters>15239.979</DistanceMeters><Cadence>72</Cadence><Extensions><TPX xmlns=\"http://www.garmin.com/xmlschemas/ActivityExtension/v2\"><Watts>231</Watts></TPX></Extensions></Trackpoint><Trackpoint><Time>2008-03-03T23:13:08Z</Time><Position><LatitudeDegrees>35.863608</LatitudeDegrees><LongitudeDegrees>-78.909587</LongitudeDegrees></Position><AltitudeMeters>74.159</AltitudeMeters><DistanceMeters>15248.820</DistanceMeters><Cadence>72</Cadence><Extensions><TPX xmlns=\"http://www.garmin.com/xmlschemas/ActivityExtension/v2\"><Watts>278</Watts></TPX></Extensions></Trackpoint><Trackpoint><Time>2008-03-03T23:13:09Z</Time><Position><LatitudeDegrees>35.863624</LatitudeDegrees><LongitudeDegrees>-78.909682</LongitudeDegrees></Position><AltitudeMeters>75.120</AltitudeMeters><DistanceMeters>15257.655</DistanceMeters><Cadence>72</Cadence><Extensions><TPX xmlns=\"http://www.garmin.com/xmlschemas/ActivityExtension/v2\"><Watts>326</Watts></TPX></Extensions></Trackpoint><Trackpoint><Time>2008-03-03T23:13:10Z</Time><Position><LatitudeDegrees>35.863640</Latitude
